vi "Calculate_Trigger_statistics.vi"(8 "Status/Errors in":refnum<vi>, 9 "Process data parameters in":T2={"Stop loop"={"Settings changed?"=FALSE, "Stop?"=refnum}, "Button refs"={"Stop program"=refnum, "Save settings"=refnum, "DAQ mode"=refnum, "Reset settings"=refnum, "Apply settings"=refnum, "Reset MAS"=refnum, "Reset SLV"=refnum, "Local DBase?"=refnum, "Last value DBase"=FALSE, "Database"=refnum, "Calibration"=refnum, "Save settings 2"=refnum}, "Process messages"={"Process message mode"=enum."Error", "Slave data?"=FALSE, "Length get settings message"=0, "Delta time"=0.0, "Data_Filter"={"Filter_Data"=FALSE, "Use_Thresh"=FALSE, "Reduce data?"=FALSE}, "Time_difference_stack"=[], "Starting sec"=0, "Ending sec"=0, "Ending sec 2"=0, "MAS_Page_Thresh"=refnum, "SLV_Page_Thresh"=refnum, "Database"=refnum}, "Settings state"={"MAS locked?"=refnum, "SLV locked?"=refnum}, "Mode"={"Mode"=enum."Dialog", "Expert?"=FALSE, "Dialog?"=FALSE}, "Alignment parameters"=refnum, "Timer parameters"=refnum, "Files"={"Path config file"=path "", "Path def. ini file"=path "", "Path ini file 1"=path "", "Path ini file 2"=path "", "Path RBF file"=path ""}, "Time difference"=refnum, "Alignment"={"GEN_Page_Calibrate"=refnum, "MAS_Page_Gain"=refnum, "MAS_Page_Offset"=refnum, "SLV_Page_Gain"=refnum, "SLV_Page_Offset"=refnum, "MAS_Page_Common"=refnum, "SLV_Page_Common"=refnum}, "Page Statistics"=refnum}, 10 "Time":dbl, 11 "GPS timestamp in":T1) -> (0 "Status/Errors out":refnum<vi>, 1 "Trigger rate /s":dbl, 2 "Process data parameters out":T2={"Stop loop"={"Settings changed?"=FALSE, "Stop?"=refnum}, "Button refs"={"Stop program"=refnum, "Save settings"=refnum, "DAQ mode"=refnum, "Reset settings"=refnum, "Apply settings"=refnum, "Reset MAS"=refnum, "Reset SLV"=refnum, "Local DBase?"=refnum, "Last value DBase"=FALSE, "Database"=refnum, "Calibration"=refnum, "Save settings 2"=refnum}, "Process messages"={"Process message mode"=enum."Error", "Slave data?"=FALSE, "Length get settings message"=0, "Delta time"=0.0, "Data_Filter"={"Filter_Data"=FALSE, "Use_Thresh"=FALSE, "Reduce data?"=FALSE}, "Time_difference_stack"=[], "Starting sec"=0, "Ending sec"=0, "Ending sec 2"=0, "MAS_Page_Thresh"=refnum, "SLV_Page_Thresh"=refnum, "Database"=refnum}, "Settings state"={"MAS locked?"=refnum, "SLV locked?"=refnum}, "Mode"={"Mode"=enum."Dialog", "Expert?"=FALSE, "Dialog?"=FALSE}, "Alignment parameters"=refnum, "Timer parameters"=refnum, "Files"={"Path config file"=path "", "Path def. ini file"=path "", "Path ini file 1"=path "", "Path ini file 2"=path "", "Path RBF file"=path ""}, "Time difference"=refnum, "Alignment"={"GEN_Page_Calibrate"=refnum, "MAS_Page_Gain"=refnum, "MAS_Page_Offset"=refnum, "SLV_Page_Gain"=refnum, "SLV_Page_Offset"=refnum, "MAS_Page_Common"=refnum, "SLV_Page_Common"=refnum}, "Page Statistics"=refnum}, 3 "GPS timestamp out":T1)   [LabVIEW 2013]
uses:
  Controls/Process_Data_Parameters.ctl
  Controls/Stop_Loop.ctl
  Controls/Button_Refs.ctl
  Controls/Process_Messages.ctl
  Controls/Process_Message_Mode.ctl
  Controls/Settings_State.ctl
  Controls/Mode.ctl
  Controls/Files.ctl
  Controls/Page_Calibration.ctl
  Controls/GPS_Timestamp.ctl
  Controls/Get_Set_Statistics_Options.ctl
  Controls/Get_Set_Statistics_Options2.ctl
  <vilib>/Utility/miscctls.llb/LVDateTimeRec.ctl
panel:
  out "unsigned 64bit integer":u64
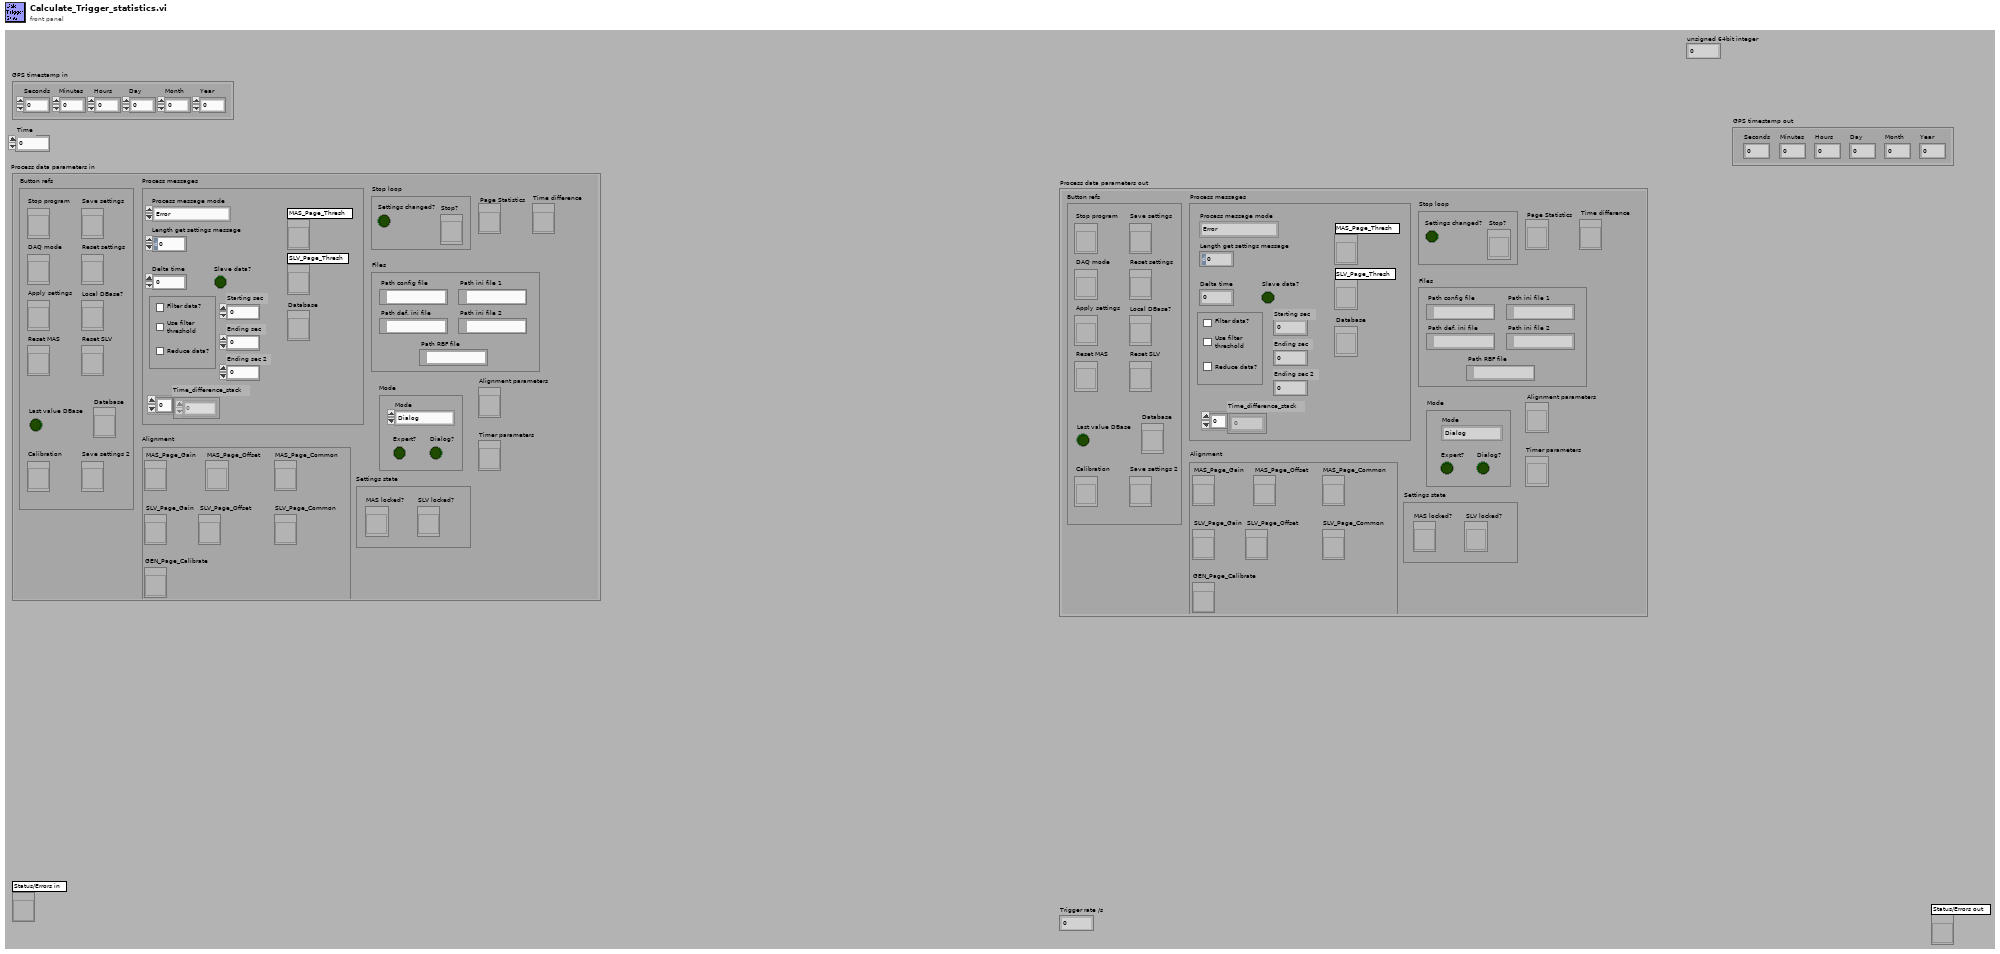
[diagram p1: front panel]
types:
  T1 = typedef "GPS_Timestamp.ctl" = cluster{"Seconds":u8, "Minutes":u8, "Hours":u8, "Day":u8, "Month":u8, "Year":u16}
  T2 = typedef "Process_Data_Parameters.ctl" = cluster{"Stop loop":T3, "Button refs":T4, "Process messages":T5, "Settings state":T7, "Mode":T8, "Alignment parameters":refnum<vi>, "Timer parameters":refnum<vi>, "Files":T9, "Time difference":refnum<vi>, "Alignment":T10, "Page Statistics":refnum<vi>}
  T3 = typedef "Stop_Loop.ctl" = cluster{"Settings changed?":bool, "Stop?":refnum<vi>}
  T4 = typedef "Button_Refs.ctl" = cluster{"Stop program":refnum<vi>, "Save settings":refnum<vi>, "DAQ mode":refnum<vi>, "Reset settings":refnum<vi>, "Apply settings":refnum<vi>, "Reset MAS":refnum<vi>, "Reset SLV":refnum<vi>, "Local DBase?":refnum<vi>, "Last value DBase":bool, "Database":refnum<vi>, "Calibration":refnum<vi>, "Save settings 2":refnum<vi>}
  T5 = typedef "Process_Messages.ctl" = cluster{"Process message mode":T6, "Slave data?":bool, "Length get settings message":i32, "Delta time":dbl, "Data_Filter":cluster{"Filter_Data":bool, "Use_Thresh":bool, "Reduce data?":bool}, "Time_difference_stack":u64[], "Starting sec":u64, "Ending sec":u64, "Ending sec 2":u64, "MAS_Page_Thresh":refnum<vi>, "SLV_Page_Thresh":refnum<vi>, "Database":refnum<vi>}
  T6 = typedef "Process_Message_Mode.ctl" = enum16{"Error", "Measurement data", "Comparator data", "One Second"}
  T7 = typedef "Settings_State.ctl" = cluster{"MAS locked?":refnum<vi>, "SLV locked?":refnum<vi>}
  T8 = typedef "Mode.ctl" = cluster{"Mode":enum8{"Stop", "Dialog", "Hisparc II", "Hisparc II DAQ", "Alignment"}, "Expert?":bool, "Dialog?":bool}
  T9 = typedef "Files.ctl" = cluster{"Path config file":path, "Path def. ini file":path, "Path ini file 1":path, "Path ini file 2":path, "Path RBF file":path}
  T10 = typedef "Page_Calibration.ctl" = cluster{"GEN_Page_Calibrate":refnum<vi>, "MAS_Page_Gain":refnum<vi>, "MAS_Page_Offset":refnum<vi>, "SLV_Page_Gain":refnum<vi>, "SLV_Page_Offset":refnum<vi>, "MAS_Page_Common":refnum<vi>, "SLV_Page_Common":refnum<vi>}
  T11 = typedef "LVDateTimeRec.ctl" = cluster{"fractional second":dbl, "second":i32, "minute":i32, "hour":i32, "day of month":i32, "month":i32, "year":i32, "day of week":i32, "day of year":i32, "DST":i32}
  T12 = typedef "Get_Set_Statistics_Options.ctl" = enum16{"Get", "Set singles", "Set events"}
  T13 = typedef "Get_Set_Statistics_Options2.ctl" = enum16{"Get", "Set"}
  T14 = cluster{"Last trigger":u64, "Time difference":u64}
  T15 = cluster{"Seconds":i32, "Minutes":i32, "Hours":i32, "Day":i32, "Month":i32, "Year":i32}
  T16 = typedef "TabPage_Statistics.ctl" = cluster{"Thresh_Count_MAS":T17, "Thresh_Count_SLV":T17, "Count":bool, "Time_to_count":u32, "Time":u32, "Time_to_count_ref":refnum<vi>, "Counting?":bool, "Baseline_MAS_Ch1":i16, "Baseline_MAS_Ch2":i16, "Baseline_SLV_Ch1":i16, "Baseline_SLV_Ch2":i16, "Basel_Err_MAS_Ch1":u32, "Basel_Err_MAS_Ch2":u32, "Basel_Err_SLV_Ch1":u32, "Basel_Err_SLV_Ch2":u32, "Peaks_Overshoot":dbl, "Height_Overshoot":dbl, "Integrals_Overshoot":dbl, "Last_event":dbl, "Total_Trigger":u32, "Av_Trigger":dbl, "Number of peaks":cluster{"t0":i32, "dt":i32, "Histogram":i32[][]}, "Pulse height":cluster{"t0":i32, "dt":i32, "Histogram":i32[][]}, "Integral":cluster{"t0":i32, "dt":i32, "Histogram":i32[][]}, "Number of peaks Entries":u64, "Number of peaks Overshoots":u64, "Pulse height  Entries":u64, "Pulse height Overshoots":u64, "Integral Entries":u64, "Integral Overshoots":u64, "Last trigger Stack":refnum<vi>}
  T17 = typedef "Page_Thresholds.ctl" = cluster{"Sing_Ch1_low":u32, "Sing_Ch1_high":u32, "Sing_Ch2_low":u32, "Sing_Ch2_high":u32, "Total_Ch1_low":u32, "Total_Ch1_high":u32, "Total_Ch2_low":u32, "Total_Ch2_high":u32, "Av_Ch1_low":dbl, "Av_Ch1_high":dbl, "Av_Ch2_low":dbl, "Av_Ch2_high":dbl}
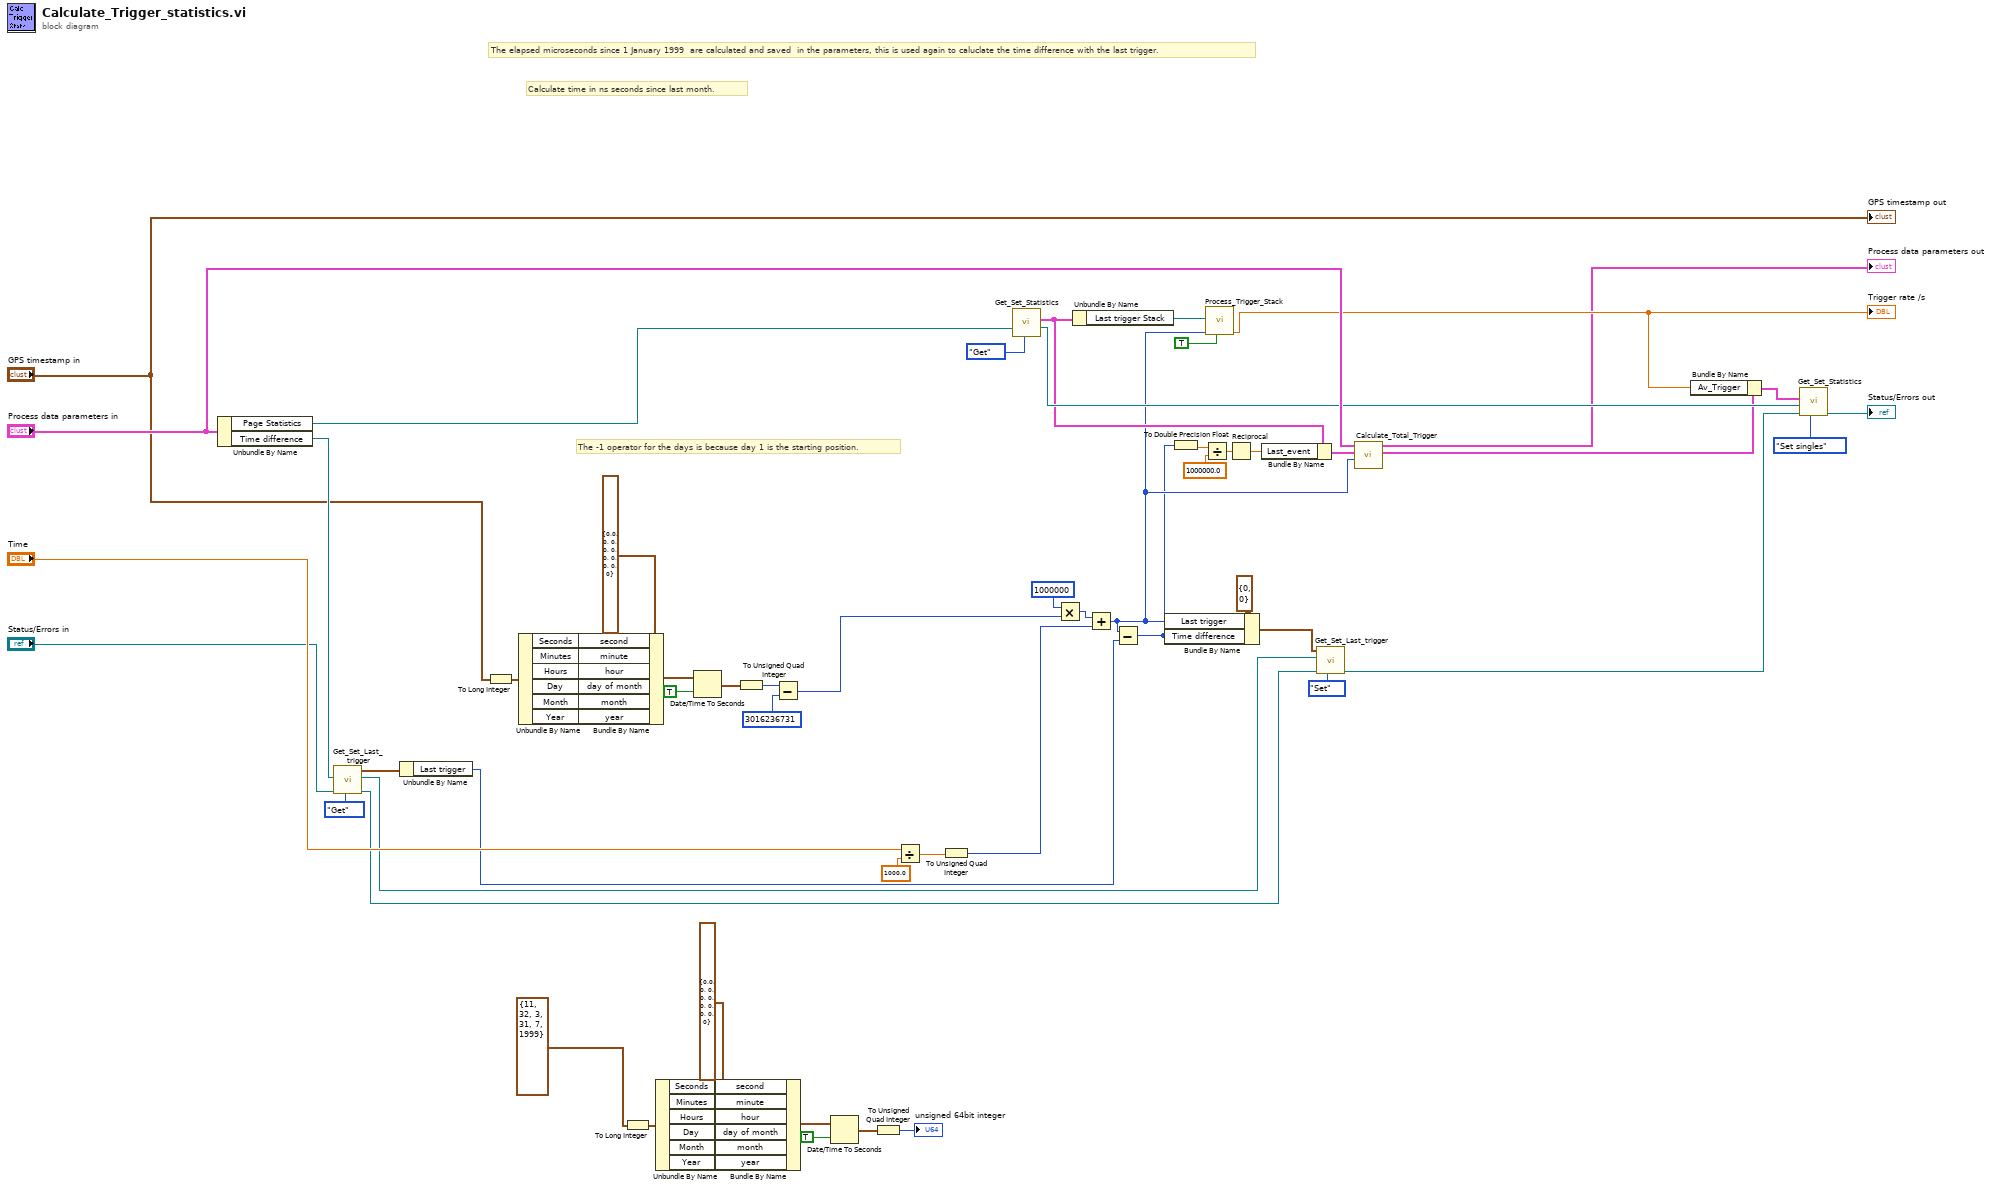
[diagram p0: block diagram]
diagram:
  # "The -1 operator for the days is because day 1 is the starting position."
  # "The elapsed microseconds since 1 January 1999  are calculated and saved  in the parameters, this is used again to caluclate the time difference with the last trigger."
  # "Calculate time in ns seconds since last month."
  n1 = Unbundle By Name("Process data parameters in") -> ("Page Statistics"=w38:refnum<vi>, "Time difference"=w56:refnum<vi>)
  n2 = call "Get_Set_Last_trigger.vi"("Get/Set"=Get_Set_Statistics_Options2."Get", "Status/Errors in"="Status/Errors in", "Time difference"=w56) -> ("Status/Errors out"=w52:refnum<vi>, "Time difference out"=w54:refnum<vi>, "Value out"=w46:T14)  [unwired: 1 in, 5 out]
  n3 = Unbundle By Name(w46) -> ("Last trigger"=w45:u64)
  n4 = To Long Integer(number="GPS timestamp in") -> (32bit integer=w27:T15)
  n5 = Unbundle By Name(w27) -> ("Seconds"=w33:i32, "Minutes"=w32:i32, "Hours"=w31:i32, "Day"=w30:i32, "Month"=w29:i32, "Year"=w28:i32)
  n6 = Bundle By Name(cluster=T11 {"fractional second"=0.0, "second"=0, "minute"=0, "hour"=0, "day of month"=0, "month"=0, "year"=0, "day of week"=0, "day of year"=0, "DST"=0} ("date time rec"), "second"=w33, "minute"=w32, "hour"=w31, "day of month"=w30, "month"=w29, "year"=w28) -> (w36:T11)
  n7 = To Long Integer(number=T1 {"Seconds"=11, "Minutes"=32, "Hours"=3, "Day"=31, "Month"=7, "Year"=1999} ("GPS timestamp in")) -> (32bit integer=w15:T15)
  n8 = Unbundle By Name(w15) -> ("Seconds"=w21:i32, "Minutes"=w20:i32, "Hours"=w19:i32, "Day"=w18:i32, "Month"=w17:i32, "Year"=w16:i32)
  n9 = Date/Time To Seconds(1:TRUE ("is UTC (F)"), 2:w36) -> (0:w26:timestamp)
  n10 = Bundle By Name(cluster=T11 {"fractional second"=0.0, "second"=0, "minute"=0, "hour"=0, "day of month"=0, "month"=0, "year"=0, "day of week"=0, "day of year"=0, "DST"=0} ("date time rec"), "second"=w21, "minute"=w20, "hour"=w19, "day of month"=w18, "month"=w17, "year"=w16) -> (w23:T11)
  n11 = To Unsigned Quad Integer(1:w26) -> (0:w10:u64)
  n12 = Subtract(x=w10, y=u64 3016236731) -> (x-y=w9:u64)
  n13 = Date/Time To Seconds(1:TRUE ("is UTC (F)"), 2:w23) -> (0:w14:timestamp)
  n14 = To Unsigned Quad Integer(1:w14) -> (0:→"unsigned 64bit integer":u64)
  n15 = Divide(x="Time", y=1000.0 ("x")) -> (x/y=w48:dbl)
  n16 = To Unsigned Quad Integer(1:w48) -> (0:w47:u64)
  n17 = call "Get_Set_Statistics.vi"("Page Statistics in"=w38, "Get/Set"=Get_Set_Statistics_Options."Get") -> ("Value out"=w7:T16, "Page Statistics out"=w37:refnum<vi>)  [unwired: 3 in, 4 out]
  n18 = Multiply(x=u64 1000000, y=w9) -> (x*y=w64:u64)
  n19 = Unbundle By Name(w7) -> ("Last trigger Stack"=w6:refnum<vi>)
  n20 = Add(x=w64, y=w47) -> (x+y=w2:u64)
  n21 = Subtract(x=w2, y=w45) -> (x-y=w1:u64)
  n22 = Bundle By Name(cluster=T14 {"Last trigger"=0, "Time difference"=0} ("input cluster"), "Last trigger"=w2, "Time difference"=w1) -> (w55:T14)
  n23 = To Double Precision Float(number=w1) -> (double precision float=w43:dbl)
  n24 = Divide(x=w43, y=1000000.0) -> (x/y=w41:dbl)
  n25 = call "Process_Trigger_Stack.vi"("Add trigger?"=TRUE, "Time"=w2, "Last trigger Stack 2"=w6) -> ("Average Trigger"=w5:dbl)  [unwired: 8 out]
  "Trigger rate /s" <- w5
  n26 = Reciprocal(x=w41) -> (1/x=w44:dbl)
  n27 = Bundle By Name(cluster=w7, "Last_event"=w44) -> (w40:T16)
  n28 = call "Get_Set_Last_trigger.vi"("Get/Set"=Get_Set_Statistics_Options2."Set", "Status/Errors in"=w52, "Time difference"=w54, "Value in"=w55) -> ("Status/Errors out"=w50:refnum<vi>)  [unwired: 7 out]
  n29 = call "Calculate_Total_Trigger.vi"("Last trigger"=w2, "Page statistics in"=w40, "Process data parameters in"="Process data parameters in") -> ("Page statistics out"=w24:T16, "Process data parameters out"=→"Process data parameters out":T2)  [unwired: 7 out]
  n30 = Bundle By Name(cluster=w24, "Av_Trigger"=w5) -> (w61:T16)
  n31 = call "Get_Set_Statistics.vi"("Value in"=w61, "Page Statistics in"=w37, "Status/Errors in"=w50, "Get/Set"=Get_Set_Statistics_Options."Set singles") -> ("Status/Errors out"=→"Status/Errors out":refnum<vi>)  [unwired: 6 out]
  "GPS timestamp out" <- "GPS timestamp in"
